vi "Finish.vi"   [LabVIEW 2016]
doc: "This VI is called just before exiting. It is expected to close I/O refnum, save collected data, etc."
uses:
  <vilib>/Rock Robotics/WPI/Utilities/WPI_GetSetVariantRefNum.vi
types:
  T1 = typedef "WPI_AnalogChannelDevRef.ctl" = cluster{"DevStatus":errorcluster, "Analog Channel":T2}
  T2 = typedef "FPGA_AIChannel.ctl" = enum8{"AI 0", "AI 1", "AI 2", "AI 3", "AI MXP 0", "AI MXP 1", "AI MXP 2", "AI MXP 3", "Invalid"}
  T3 = typedef "WPI_SolenoidDevRef.ctl" = cluster{"DevStatus":errorcluster, "Pneumatics Control Module":u8, "Forward Solenoid Channel":T4, "Reverse Solenoid Channel":T4}
  T4 = typedef "WPI_SolenoidChannel.ctl" = enum8{"Solenoid 0", "Solenoid 1", "Solenoid 2", "Solenoid 3", "Solenoid 4", "Solenoid 5", "Solenoid 6", "Solenoid 7", "Invalid"}
  T5 = typedef "WPI_MotorControlDeviceRef.ctl" = cluster{"DeviceStatus":errorcluster, "Type":T6, "PWM":cluster{"PWM Channel":T7, "DeadBand":T8}, "CAN":cluster{"Device Number":u8, "SetOutput VI Ref":variant, "GetOutput VI Ref":variant, "Enable VI Ref":variant, "Disable VI Ref":variant, "Data":variant}, "Invert":bool}
  T6 = typedef "WPI_MotorControlType.ctl" = enum16{"PWM", "CAN"}
  T7 = typedef "FPGA_DIOPWMChannel.ctl" = enum8{"PWM 0", "PWM 1", "PWM 2", "PWM 3", "PWM 4", "PWM 5", "PWM 6", "PWM 7", "PWM 8", "PWM 9", "PWM MXP 0", "PWM MXP 1", "PWM MXP 2", "PWM MXP 3", "PWM MXP 4", "PWM MXP 5", "PWM MXP 6", "PWM MXP 7", "PWM MXP 8", "PWM MXP 9", "Invalid"}
  T8 = typedef "WPI_PWMDeadband.ctl" = cluster{"Name":string, "maxPositivePwm":i32, "minPositivePwm":i32, "centerPwm":i32, "maxNegativePwm":i32, "minNegativePwm":i32, "angularRange":u16}
  T9 = typedef "WPI_JoystickDevRef.ctl" = cluster{"Device":T10}
  T10 = typedef "WPI_JoystickDeviceEnum.ctl" = enum16{"USB 0", "USB 1", "USB 2", "USB 3", "USB 4", "USB 5"}
  T11 = typedef "WPI_RobotDriveDevRef.ctl" = cluster{"DevStatus":errorcluster, "Motors[]":T5[], "Square Inputs":bool, "Max Output":dbl}
  T12 = typedef "WPI_CompressorDevRef.ctl" = cluster{"DevStatus":errorcluster, "Pneumatics Control Module":u8}
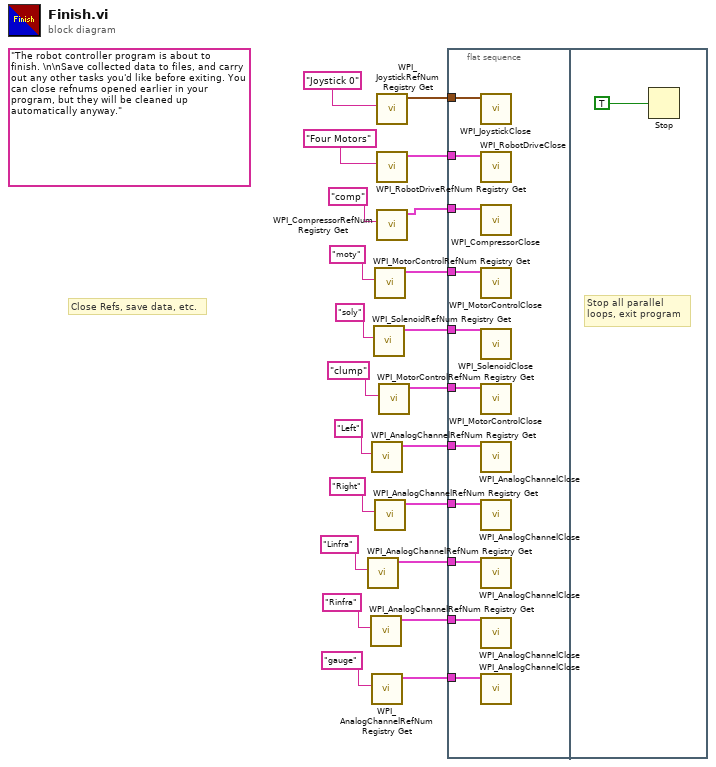
[diagram p0: block diagram]
diagram:
  (unwired) "The robot controller program is about to finish. \n\nSave collected data to files, and carry out any other tasks you'd like before exiting. You can close refnums opened earlier in your program, but they will be cleaned up automatically anyway."
  # "Close Refs, save data, etc."
  n1 = call <vilib>:"WPI_AnalogChannelRefNum Registry Get.vi"("refnum name"="Linfra") -> ("AIDeviceRef"=w3:T1)  [unwired: 9 in, 1 out]
  n2 = call <vilib>:"WPI_AnalogChannelRefNum Registry Get.vi"("refnum name"="Rinfra") -> ("AIDeviceRef"=w1:T1)  [unwired: 9 in, 1 out]
  n3 = call <vilib>:"WPI_AnalogChannelRefNum Registry Get.vi"("refnum name"="Left") -> ("AIDeviceRef"=w5:T1)  [unwired: 9 in, 1 out]
  n4 = call <vilib>:"WPI_AnalogChannelRefNum Registry Get.vi"("refnum name"="gauge") -> ("AIDeviceRef"=w2:T1)  [unwired: 9 in, 1 out]
  n5 = call <vilib>:"WPI_SolenoidRefNum Registry Get.vi"("refnum name"="soly") -> ("SolenoidDevRef"=w6:T3)  [unwired: 9 in, 1 out]
  n6 = call <vilib>:"WPI_MotorControlRefNum Registry Get.vi"("refnum name"="moty") -> ("MotorControlDevRef"=w8:T5)  [unwired: 9 in, 1 out]
  n7 = call <vilib>:"WPI_AnalogChannelRefNum Registry Get.vi"("refnum name"="Right") -> ("AIDeviceRef"=w4:T1)  [unwired: 9 in, 1 out]
  n8 = call <vilib>:"WPI_JoystickRefNum Registry Get.vi"("refnum name"="Joystick 0") -> ("JoystickDevRef"=w19:T9)  [unwired: 1 in, 9 out]
  n9 = call <vilib>:"WPI_RobotDriveRefNum Registry Get.vi"("refnum name"="Four Motors") -> ("RobotDriveDevRef"=w20:T11)  [unwired: 1 in, 9 out]
  n10 = call <vilib>:"WPI_CompressorRefNum Registry Get.vi"("refnum name"="comp") -> ("CompressorDevRef"=w9:T12)  [unwired: 9 in, 1 out]
  n11 = call <vilib>:"WPI_MotorControlRefNum Registry Get.vi"("refnum name"="clump") -> ("MotorControlDevRef"=w7:T5)  [unwired: 9 in, 1 out]
  n12 = flat-sequence {
    tunnel: w20 -> [w33]
    tunnel: w19 -> [w32]
    tunnel: w9 -> [w31]
    tunnel: w8 -> [w30]
    tunnel: w7 -> [w29]
    tunnel: w6 -> [w28]
    tunnel: w5 -> [w27]
    tunnel: w4 -> [w26]
    tunnel: w3 -> [w25]
    tunnel: w2 -> [w24]
    tunnel: w1 -> [w23]
    frame #0 {
      n13 = call <vilib>:"WPI_JoystickClose.vi"("JoystickDevRef"=w32) -> ()  [unwired: 11 out]
      n14 = call <vilib>:"WPI_RobotDriveClose.vi"("RobotDriveDevRef"=w33) -> ()  [unwired: 1 in, 10 out]
      n15 = call <vilib>:"WPI_CompressorClose.vi"("CompressorDevRef"=w31) -> ()  [unwired: 10 in, 1 out]
      n16 = call <vilib>:"WPI_MotorControlClose.vi"("MotorControlDevRef"=w30) -> ()  [unwired: 10 in, 1 out]
      n17 = call <vilib>:"WPI_SolenoidClose.vi"("SolenoidDevRef"=w28) -> ()  [unwired: 10 in, 1 out]
      n18 = call <vilib>:"WPI_MotorControlClose.vi"("MotorControlDevRef"=w29) -> ()  [unwired: 10 in, 1 out]
      n19 = call <vilib>:"WPI_AnalogChannelClose.vi"("AIDeviceRef"=w27) -> ()  [unwired: 10 in, 1 out]
      n20 = call <vilib>:"WPI_AnalogChannelClose.vi"("AIDeviceRef"=w26) -> ()  [unwired: 10 in, 1 out]
      n21 = call <vilib>:"WPI_AnalogChannelClose.vi"("AIDeviceRef"=w25) -> ()  [unwired: 10 in, 1 out]
      n22 = call <vilib>:"WPI_AnalogChannelClose.vi"("AIDeviceRef"=w23) -> ()  [unwired: 10 in, 1 out]
      n23 = call <vilib>:"WPI_AnalogChannelClose.vi"("AIDeviceRef"=w24) -> ()  [unwired: 10 in, 1 out]
    }
    frame #1 {
      # "Stop all parallel\nloops, exit program"
      n24 = Stop(stop? (T)=TRUE ("Quit")) -> ()
    }
  }
